vi "testing odor and manifold configuration.vi"() -> ()   [LabVIEW 2021]
uses:
  type-defs/manifold configuration cluster (type def).ctl
  type-defs/manifold selection.ctl
  type-defs/single port single odor cluster.ctl
  type-defs/port number (type def).ctl
  type-defs/odor selection (type def).ctl
  type-defs/odor color (type def).ctl
  type-defs/odor description array (type def).ctl
  type-defs/odor info cluster (type def).ctl
panel:
  in  "odor descriptions":T1
  in  "stimulator connections":T5[](array[typedef])
  in  "num stimulator ports":i32
  in  "stop":bool
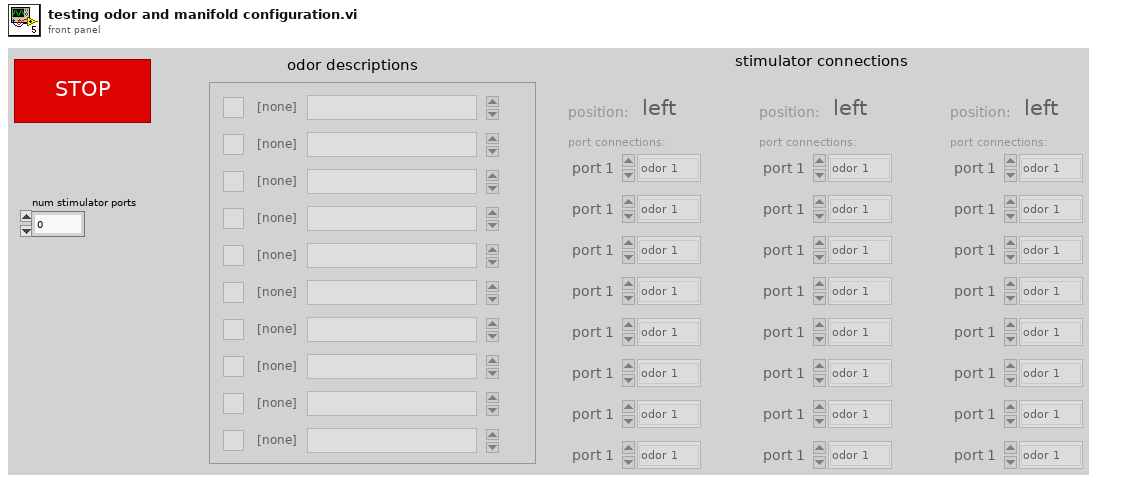
[diagram p1: front panel]
types:
  T1 = typedef "odor description array (type def).ctl" = T2[]
  T2 = typedef "odor info cluster (type def).ctl" = cluster{"odor channel":T3, "odor description":string, "odor color":T4, "odor channel active":bool}
  T3 = typedef "odor selection (type def).ctl" = enum16{"[none]", "odor 1", "odor 2", "odor 3", "odor 4", "odor 5", "odor 6", "odor 7", "odor 8", "odor 9", "odor 10"}
  T4 = typedef "odor color (type def).ctl" = u16
  T5 = typedef "manifold configuration cluster (type def).ctl" = cluster{"position:":T6, "port connections:":T7[]}
  T6 = typedef "manifold selection.ctl" = enum16{"left", "middle", "right"}
  T7 = typedef "single port single odor cluster.ctl" = cluster{"port number":T8, "connected odor":T3, "error":bool, "odor color":T4}
  T8 = typedef "port number (type def).ctl" = enum16{"port 1", "port 2", "port 3", "port 4", "port 5", "port 6", "port 7", "port 8"}
  T9 = enum8{"Enabled", "Disabled", "Disabled and Grayed Out"}
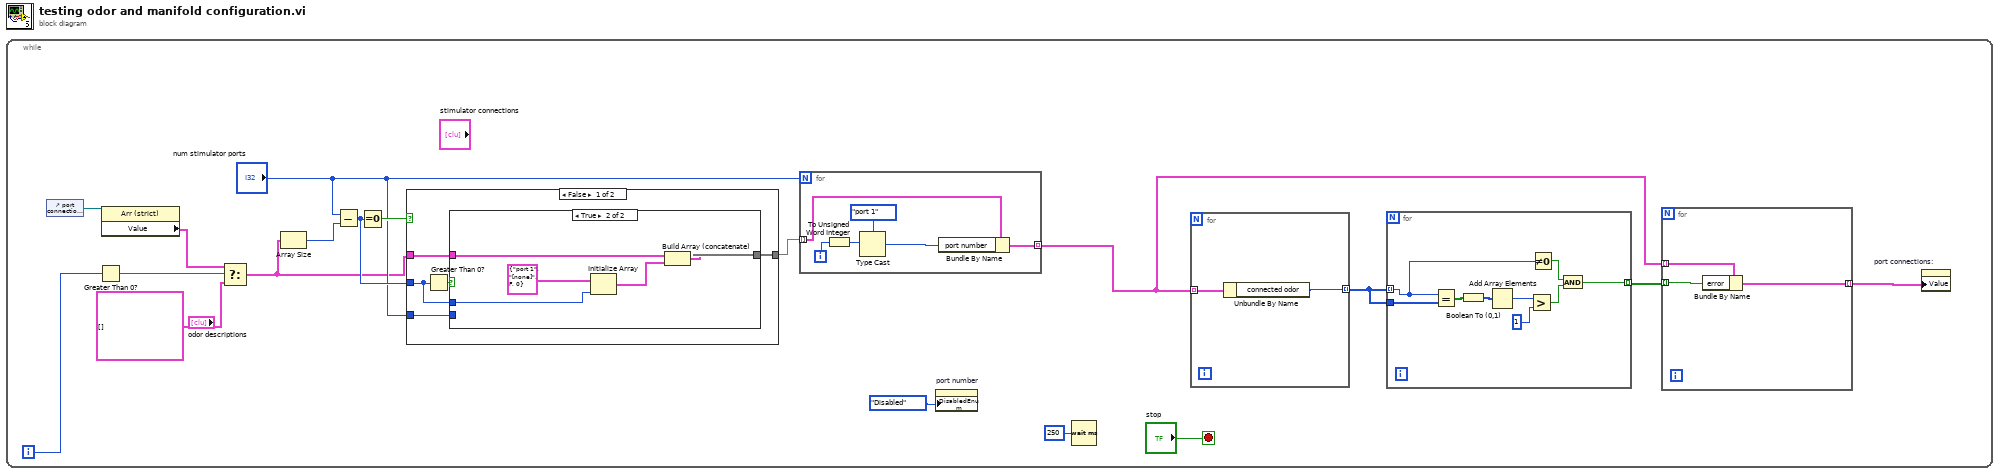
[diagram p0: block diagram]
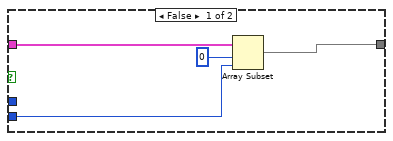
[diagram p2: hidden frame]
diagram:
  n1 = while {
    i -> [w10]
    stop <- "stop" stop-if-true
    n2 = control-ref of="port connections:"() -> (w1:refnum<vi>)
    n3 = Greater Than 0?(x=w10) -> (x > 0?=w9:bool)
    n4 = property on="Property Node" class="Arr (strict)"(reference=w1) -> ("Value"=w2:T7[])  [unwired: 1 in, 2 out]
    n5 = Select(t=w2, s=w9, f=T7[] [] ("Value")) -> (s? t:f=w8:T7[])
    n6 = Array Size(array=w8) -> (size(s)=w16:i32)
    n7 = Subtract(x="num stimulator ports", y=w16) -> (x-y=w13:i32)
    n8 = Equal To 0?(x=w13) -> (x = 0?=w14:bool)
    n9 = case shown="False" w14 {
      tunnel: w8 -> [w36 w47]
      tunnel: [w35 w47] -> w15
      tunnel: w13 -> [w33 _]
      tunnel: "num stimulator ports" -> [w34 _]
      frame False {
        n10 = Greater Than 0?(x=w33) -> (x > 0?=w37:bool)
        n11 = case shown="True" w37 {
          tunnel: w33 -> [_ w46]
          tunnel: w36 -> [w41 w45]
          tunnel: [w39 w44] -> w35
          tunnel: w34 -> [w38 _]
          frame False {
            n12 = Array Subset(array=w41, index=0, length=w38) -> (w39:T7[])
          }
          frame True {
            n13 = Initialize Array(T7 {"port number"=enum."port 1", "connected odor"=enum."[none]", "error"=FALSE, "odor color"=0} ("port-odor cluster"), w46) -> (w42:T7[])
            n14 = Build Array (concatenate)(w45, w42) -> (w44:T7[])
          }
        }
      }
      frame True {
      }
    }
    n15 = for {
      N: "num stimulator ports" -> [_]
      tunnel: [w51] -> w3 mode=indexing
      tunnel: w15 -> [w50] mode=indexing
      i -> [w53]
      n16 = To Unsigned Word Integer(number=w53) -> (unsigned 16bit integer=w49:u16)
      n17 = Type Cast(type=port_number_(type_def)."port 1" ("port number"), x=w49) -> (*(type *) &x=w48:T8)
      n18 = Bundle By Name(cluster=w50, "port number"=w48) -> (w51:T7)
    }
    n19 = property on="port number" class="Enum (strict)"("DisabledEnum"=T9."Disabled" ("Disabled")) -> ()  [unwired: 2 in, 2 out]
    n20 = Wait (ms)(milliseconds to wait=u32 250) -> ()  [unwired: 1 out]
    n21 = for {
      tunnel: w3 -> [w32] mode=indexing
      tunnel: [w31] -> w7 mode=indexing
      n22 = Unbundle By Name(w32) -> ("connected odor"=w31:T3)
    }
    n23 = for {
      tunnel: w7 -> [w25] mode=indexing
      tunnel: w7 -> [w30]
      tunnel: [w22] -> w5 mode=indexing
      n24 = Equal?(x=w25, y=w30) -> (x = y?=w29:bool[])
      n25 = Boolean To (0,1)(Boolean=w29) -> (0, 1=w28:i16[])
      n26 = Add Array Elements(numeric array=w28) -> (sum=w27:i16)
      n27 = Greater?(x=w27, y=i16 1) -> (0:w24:bool)
      n28 = Not Equal To 0?(x=w25) -> (x != 0?=w23:bool)
      n29 = And(x=w23, y=w24) -> (x .and. y?=w22:bool)
    }
    n30 = for {
      tunnel: w5 -> [w20] mode=indexing
      tunnel: w3 -> [w21] mode=indexing
      tunnel: [w19] -> w4 mode=indexing
      n31 = Bundle By Name(cluster=w21, "error"=w20) -> (w19:T7)
    }
    n32 = property on="port connections:" class="Arr (strict)"("Value"=w4) -> ()  [unwired: 2 in, 2 out]
  }
